vi "test_variance_map_filtered.vi"() -> ()   [LabVIEW 2009]
doc: "Copyright (C) 2009, Stepan A. Baranov\nweb: http://www.OCTLab.org/\nemail: stepan@baranov.su"
uses:
  <vilib>/Analysis/NI_AALBase.lvlib
  OCTLib.dll
panel:
  out "min":dbl format="%0.2f"
  out "max":dbl format="%0.2f"
  out "vertical radius":i32
  out "error out":errorcluster
  out "horizontal radius":i32
  out "width":i32
  out "height":i32
  in  "Small/Big":bool
  out "loop #":i32
  out "RSM_STAT time":u32
  out "LabView time":u32
  out "RSM_STAT Array":dbl[][](array[numeric])
  out "LabView Array":dbl[][](array[numeric])
  in  "stop":bool
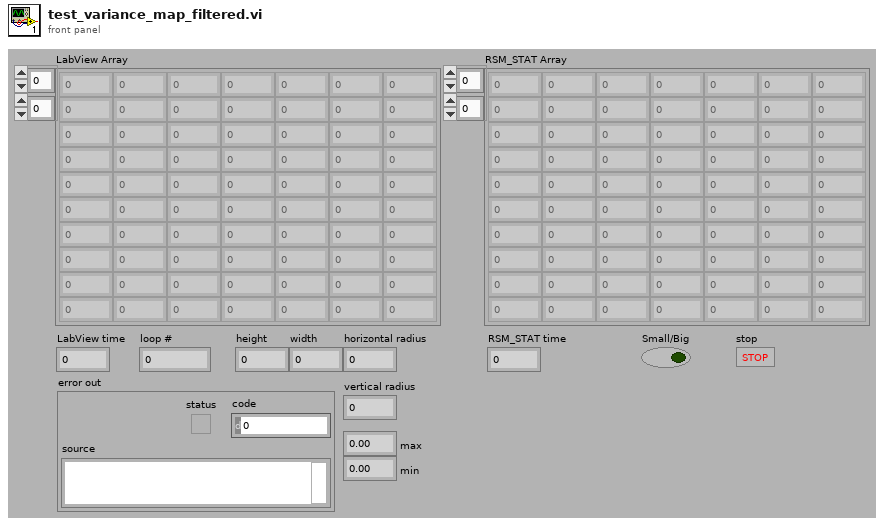
[diagram p1: front panel]
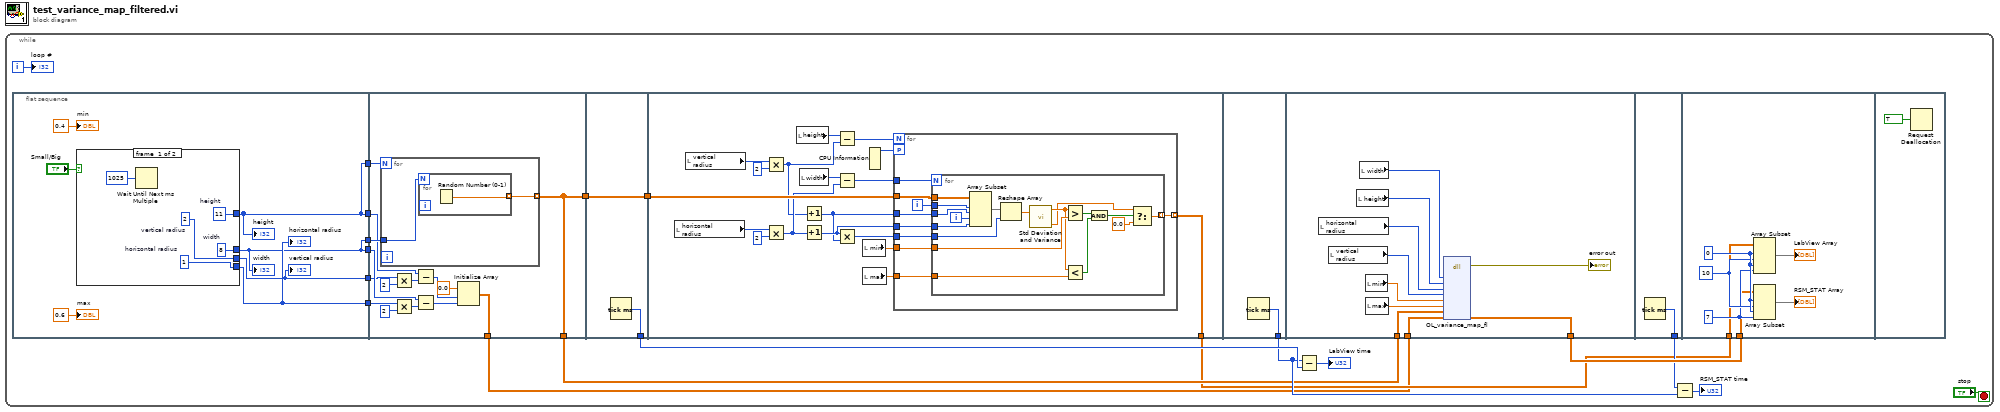
[diagram p0: block diagram]
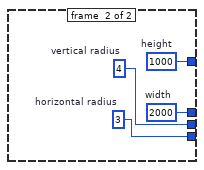
[diagram p2: hidden frame]
diagram:
  n1 = while {
    i -> [w12]
    stop <- "stop" stop-if-true
    n2 = flat-sequence {
      tunnel: [w23] -> w8
      tunnel: [w24] -> w7
      tunnel: [w25] -> w5
      tunnel: [w24] -> w4
      tunnel: [w23] -> w3
      tunnel: [w22] -> w1
      tunnel: [w48] -> w11
      tunnel: [w48] -> w9
      tunnel: w8 -> [w50]
      tunnel: w7 -> [w49]
      tunnel: w5 -> [w46]
      tunnel: w4 -> [w44]
      tunnel: w3 -> [w42]
      tunnel: [w39] -> w2
      tunnel: w1 -> [w37]
      tunnel: [w55] -> w17
      tunnel: [w54] -> w10
      tunnel: w9 -> [w54]
      tunnel: w10 -> [w73]
      tunnel: [w69] -> w6
      tunnel: [w100] -> w14
      tunnel: w11 -> [w109]
      tunnel: [w108] -> w18
      tunnel: w2 -> [w110]
      tunnel: [w111] -> w15
      tunnel: w18 -> [w114]
      tunnel: w6 -> [w113]
      frame #0 {
        n3 = case shown="False" "Small/Big" {
          tunnel: [w29 w35] -> w24
          tunnel: [w30 w34] -> w23
          tunnel: [w31 w33] -> w25
          tunnel: [w27 w32] -> w22
          frame #0 {
            w27 = 2  # vertical radius
            w31 = 1  # horizontal radius
            w30 = 8  # width
            w29 = 11  # height
            n4 = Wait Until Next ms Multiple(millisecond multiple=u32 1025) -> ()  [unwired: 1 out]
          }
          frame #1 {
            w32 = 4  # vertical radius
            w33 = 3  # horizontal radius
            w34 = 2000  # width
            w35 = 1000  # height
          }
        }
        "height" <- w24
        "width" <- w23
        "horizontal radius" <- w25
        "vertical radius" <- w22
        "max" <- 0.6 ("max")
        "min" <- 0.4 ("min")
      }
      frame #1 {
        n5 = for {
          N: w49 -> [_]
          tunnel: w50 -> [w52]
          tunnel: [w51] -> w48 mode=indexing
          n6 = for {
            N: w52 -> [_]
            tunnel: [w53] -> w51 mode=indexing
            n7 = Random Number (0-1)() -> (number: 0 to 1=w53:dbl)
          }
        }
        n8 = Multiply(x=w37, y=2) -> (x*y=w36:i32)
        n9 = Multiply(x=w46, y=2) -> (x*y=w41:i32)
        n10 = Subtract(x=w44, y=w36) -> (x-y=w43:i32)
        n11 = Subtract(x=w42, y=w41) -> (x-y=w40:i32)
        n12 = Initialize Array(0.0 ("element"), w43, w40) -> (w39:dbl[][])
      }
      frame #2 {
        n13 = Tick Count (ms)() -> (millisecond timer value=w55:u32)
      }
      frame #3 {
        n14 = local read "horizontal radius"() -> (w72:i32)
        n15 = local read "vertical radius"() -> (w61:i32)
        n16 = Multiply(x=w61, y=2) -> (x*y=w59:i32)
        n17 = Multiply(x=w72, y=2) -> (x*y=w65:i32)
        n18 = local read "height"() -> (w68:i32)
        n19 = local read "width"() -> (w66:i32)
        n20 = Increment(x=w59) -> (x+1=w58:i32)
        n21 = Increment(x=w65) -> (x+1=w60:i32)
        n22 = Subtract(x=w68, y=w59) -> (x-y=w67:i32)
        n23 = Subtract(x=w66, y=w65) -> (x-y=w64:i32)
        n24 = Multiply(x=w60, y=w58) -> (x*y=w70:i32)
        n25 = local read "min"() -> (w57:dbl)
        n26 = local read "max"() -> (w56:dbl)
        n27 = CPU Information() -> (4:w63:i32)  [unwired: 3 out]
        n28 = for {
          N: w67 -> [_]
          tunnel: w73 -> [w81]
          tunnel: w70 -> [w80]
          tunnel: [w79] -> w69 mode=indexing
          tunnel: w60 -> [w78]
          tunnel: w64 -> [w77]
          workers-P: w63 -> [_]
          tunnel: w58 -> [w76]
          tunnel: w57 -> [w75]
          tunnel: w56 -> [w74]
          i -> [w82]
          n29 = for {
            N: w77 -> [_]
            tunnel: w82 -> [w99]
            tunnel: w81 -> [w97]
            tunnel: w80 -> [w93]
            tunnel: [w86] -> w79 mode=indexing
            tunnel: w78 -> [w96]
            tunnel: w76 -> [w95]
            tunnel: w75 -> [w91]
            tunnel: w74 -> [w90]
            i -> [w98]
            n30 = Array Subset(array=w97, index (row)=w99, length (row)=w95, index (col)=w98, length (col)=w96) -> (w92:dbl[][])
            n31 = Reshape Array(w92, w93) -> (w94:dbl[])
            n32 = call <vilib>:"Std Deviation and Variance.vi"("X"=w94) -> ("mean"=w84:dbl, "variance"=w83:dbl)  [unwired: 1 in, 1 out]
            n33 = Greater?(x=w84, y=w91) -> (0:w88:bool)
            n34 = Less?(x=w84, y=w90) -> (x < y?=w89:bool)
            n35 = And(x=w88, y=w89) -> (x .and. y?=w87:bool)
            n36 = Select(t=w83, s=w87, f=0.0) -> (s? t:f=w86:dbl)
          }
        }
      }
      frame #4 {
        n37 = Tick Count (ms)() -> (millisecond timer value=w100:u32)
      }
      frame #5 {
        n38 = local read "horizontal radius"() -> (w104:i32)
        n39 = local read "vertical radius"() -> (w103:i32)
        n40 = local read "height"() -> (w106:i32)
        n41 = local read "width"() -> (w107:i32)
        n42 = local read "min"() -> (w102:dbl)
        n43 = local read "max"() -> (w101:dbl)
        n44 = dll-call lib="OCTLib.dll" fn="OL_variance_map_fl"("width"=w107, "height"=w106, "horizontal radius"=w104, "vertical radius"=w103, "min"=w102, "max"=w101, "input"=w109, "output"=w110) -> (error out=→"error out":errorcluster, "output"=w108:dbl[][])  [unwired: 11 in, 1 out]
      }
      frame #6 {
        n45 = Tick Count (ms)() -> (millisecond timer value=w111:u32)
      }
      frame #7 {
        w117 = 10 ("length")
        w116 = 7 ("length")
        w118 = 0 ("index")
        n46 = Array Subset(array=w113, index (row)=w118, length (row)=w117, index (col)=w118, length (col)=w116) -> (→"LabView Array":dbl[][])
        n47 = Array Subset(array=w114, index (row)=w118, length (row)=w117, index (col)=w118, length (col)=w116) -> (→"RSM_STAT Array":dbl[][])
      }
      frame #8 {
        n48 = Request Deallocation(TRUE ("flag")) -> ()
      }
    }
    n49 = Subtract(x=w14, y=w17) -> (x-y=→"LabView time":u32)
    n50 = Subtract(x=w15, y=w14) -> (x-y=→"RSM_STAT time":u32)
    "loop #" <- w12
  }
